vi "Teleop.vi"(10 "Match Info":T1={"Autonomous Elapsed Seconds"=0.0, "TeleOp Elapsed Seconds"=0.0, "Disabled Elapsed Seconds"=0.0, "Visited Autonomous"=FALSE, "Visited TeleOp"=FALSE, "Visited Disabled"=FALSE, "Autonomous Settings"={"Autonomous Style"=enum."Independent", "VI Refnum"=refnum}}, 11 "Call Context":T2) -> ()   [LabVIEW 2011]
doc: "This VI is called for each TeleOp packet received from the DS where the robot is not disabled. It is often used to read from the joysticks and update I/O or to update setpoints for timed control loops. It should complete and return within 20 milliseconds or it may miss DS packets."
uses:
  <vilib>/Rock Robotics/WPI/DriverStation/WPI_DriverStationDerivedRobotMode.ctl
  <vilib>/Rock Robotics/WPI/DriverStation/WPI_DriverStationMatch Info.ctl
  <vilib>/Rock Robotics/WPI/Relay/WPI_RelayValue.ctl
  <vilib>/Rock Robotics/WPI/DriverStation/DriverStationLCD/WPI_DriverStationLCDLCDLine.ctl
  Robot Global Data.vi
panel:
  in  "LDrive0":dbl
  in  "Rdrive0":dbl=0.9
  in  "Rdrive2":dbl=0.6
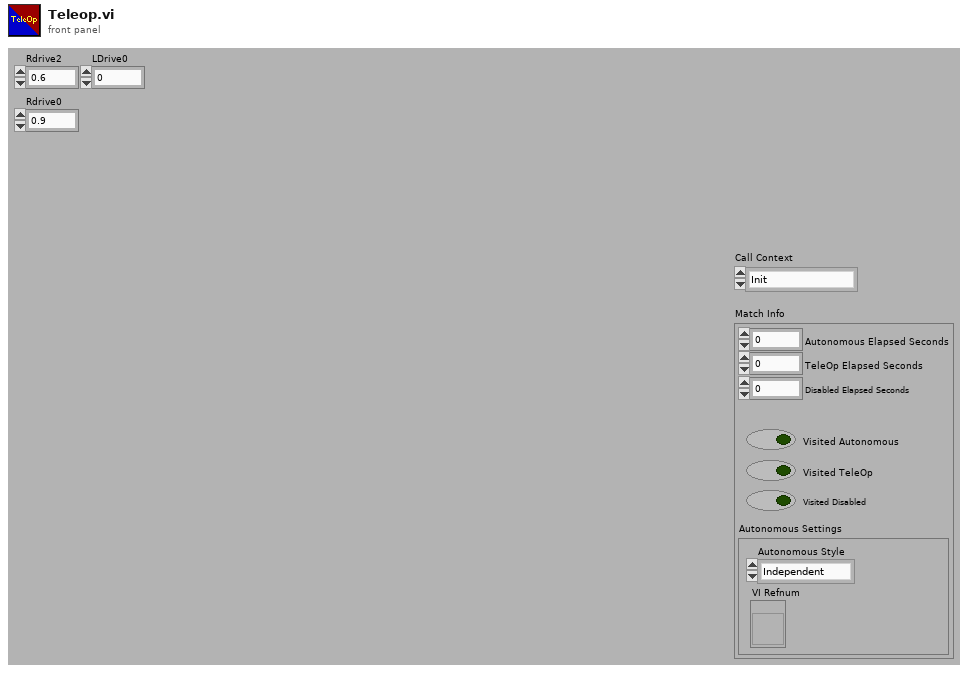
[diagram p1: front panel]
types:
  T1 = typedef "WPI_DriverStationMatch Info.ctl" = cluster{"Autonomous Elapsed Seconds":dbl, "TeleOp Elapsed Seconds":dbl, "Disabled Elapsed Seconds":dbl, "Visited Autonomous":bool, "Visited TeleOp":bool, "Visited Disabled":bool, "Autonomous Settings":cluster{"Autonomous Style":enum16{"Iterative", "Independent"}, "VI Refnum":refnum<vi>}}
  T2 = typedef "WPI_DriverStationDerivedRobotMode.ctl" = enum16{"Init", "Execute", "Stop"}
  T3 = typedef "WPI_RelayValue.ctl" = enum16{"Off", "On", "Forward", "Reverse"}
  T4 = typedef "WPI_JoystickDevRef.ctl" = cluster{"Device":T5}
  T5 = typedef "WPI_JoystickDeviceEnum.ctl" = enum16{"USB 1", "USB 2", "USB 3", "USB 4", "Kinect 1", "Kinect 2"}
  T6 = typedef "WPI_JoystickButtonState.ctl" = cluster{"Button 1":bool, "Button 2":bool, "Button 3":bool, "Button 4":bool, "Button 5":bool, "Button 6":bool, "Button 7":bool, "Button 8":bool, "Button 9":bool, "Button 10":bool, "Button 11":bool, "Button 12":bool}
  T7 = cluster{"axis 1 (x)":dbl, "axis 2 (y)":dbl, "axis 3 (throttle)":dbl, "axis 4":dbl, "axis 5":dbl, "axis 6":dbl}
  T8 = typedef "WPI_MotorControlDeviceRef.ctl" = cluster{"DeviceStatus":errorcluster, "Type":enum16{"PWM", "CAN"}, "PWM":cluster{"Digital Module":T9, "PWM Channel":T10, "DeadBand":T11}, "CAN":cluster{"Device Number":u8, "Control Mode":T12, "Semaphore":T13, "Max Vout":dbl}, "Invert":bool, "TransformRef":T14, "InvTransformRef":T14}
  T9 = typedef "FPGA_TypedefDigitalModule.ctl" = enum16{"Digital Module 1", "Digital Module 2"}
  T10 = typedef "FPGA_DIOPWMChannel.ctl" = enum8{"PWM 1", "PWM 2", "PWM 3", "PWM 4", "PWM 5", "PWM 6", "PWM 7", "PWM 8", "PWM 9", "PWM 10", "Invalid"}
  T11 = typedef "WPI_PWMDeadband.ctl" = cluster{"Name":string, "maxPositivePwm":i32, "minPositivePwm":i32, "centerPwm":i32, "maxNegativePwm":i32, "minNegativePwm":i32, "angularRange":u16}
  T12 = typedef "WPI_CANJaguar_ControlMode.ctl" = enum8{"Percent VBus", "Current", "Speed", "Position", "Voltage"}
  T13 = typedef "Semaphore RefNum" = refnum<k1>
  T14 = typedef "WPI_PWMTransform_ConPane.ctl" = refnum<vi>
  T15 = cluster{"Driver Station Digital Input (1-8)[0]":bool, "Driver Station Digital Input (1-8)[1]":bool, "Driver Station Digital Input (1-8)[2]":bool, "Driver Station Digital Input (1-8)[3]":bool, "Driver Station Digital Input (1-8)[4]":bool, "Driver Station Digital Input (1-8)[5]":bool, "Driver Station Digital Input (1-8)[6]":bool, "Driver Station Digital Input (1-8)[7]":bool, "Driver Station Digital Input (1-8)[8]":bool}
  T16 = typedef "WPI_RelayDevRef.ctl" = cluster{"DevStatus":errorcluster, "Relay Channel":T17, "Digital Module":T9, "Relay Direction":T18}
  T17 = typedef "FPGA_DIORelayChannel.ctl" = enum8{"Relay 1", "Relay 2", "Relay 3", "Relay 4", "Relay 5", "Relay 6", "Relay 7", "Relay 8", "Invalid"}
  T18 = typedef "WPI_RelayDirection.ctl" = enum16{"Both directions", "Forward only", "Reverse only"}
  T19 = typedef "WPI_DigitalInputDevRef.ctl" = cluster{"DevStatus":errorcluster, "DIO Channel":T20, "Digital Module":T9}
  T20 = typedef "FPGA_DIOChannel.ctl" = enum8{"DIO 1", "DIO 2", "DIO 3", "DIO 4", "DIO 5", "DIO 6", "DIO 7", "DIO 8", "DIO 9", "DIO 10", "DIO 11", "DIO 12", "DIO 13", "DIO 14", "Invalid"}
  T21 = typedef "WPI_EncoderDevRef.ctl" = cluster{"DevStatus":errorcluster, "EncoderIndex":T22, "CounterIndex":T23, "DistancePerCount":dbl, "Decoding Type":T24}
  T22 = typedef "FPGA_EncoderIdx.ctl" = enum8{"Enc 0", "Enc 1", "Enc 2", "Enc 3", "Invalid"}
  T23 = typedef "FPGA_CounterCtrSystemIndex.ctl" = enum8{"Ctr 0", "Ctr 1", "Ctr 2", "Ctr 3", "Ctr 4", "Ctr 5", "Ctr 6", "Ctr 7", "Invalid"}
  T24 = typedef "WPI_EncoderType.ctl" = enum16{"1x", "2x", "4x"}
  T25 = typedef "WPI_DriverStationLCDLCDLine.ctl" = enum16{"Main - Line 1", "User - Line 2", "User - Line 3", "User - Line 4", "User - Line 5", "User - Line 6"}
  T26 = typedef "WPI_ServoDeviceRef.ctl" = cluster{"DeviceStatus":errorcluster, "Digital Module":T9, "PWM Channel":T10, "DeadBand":T11}
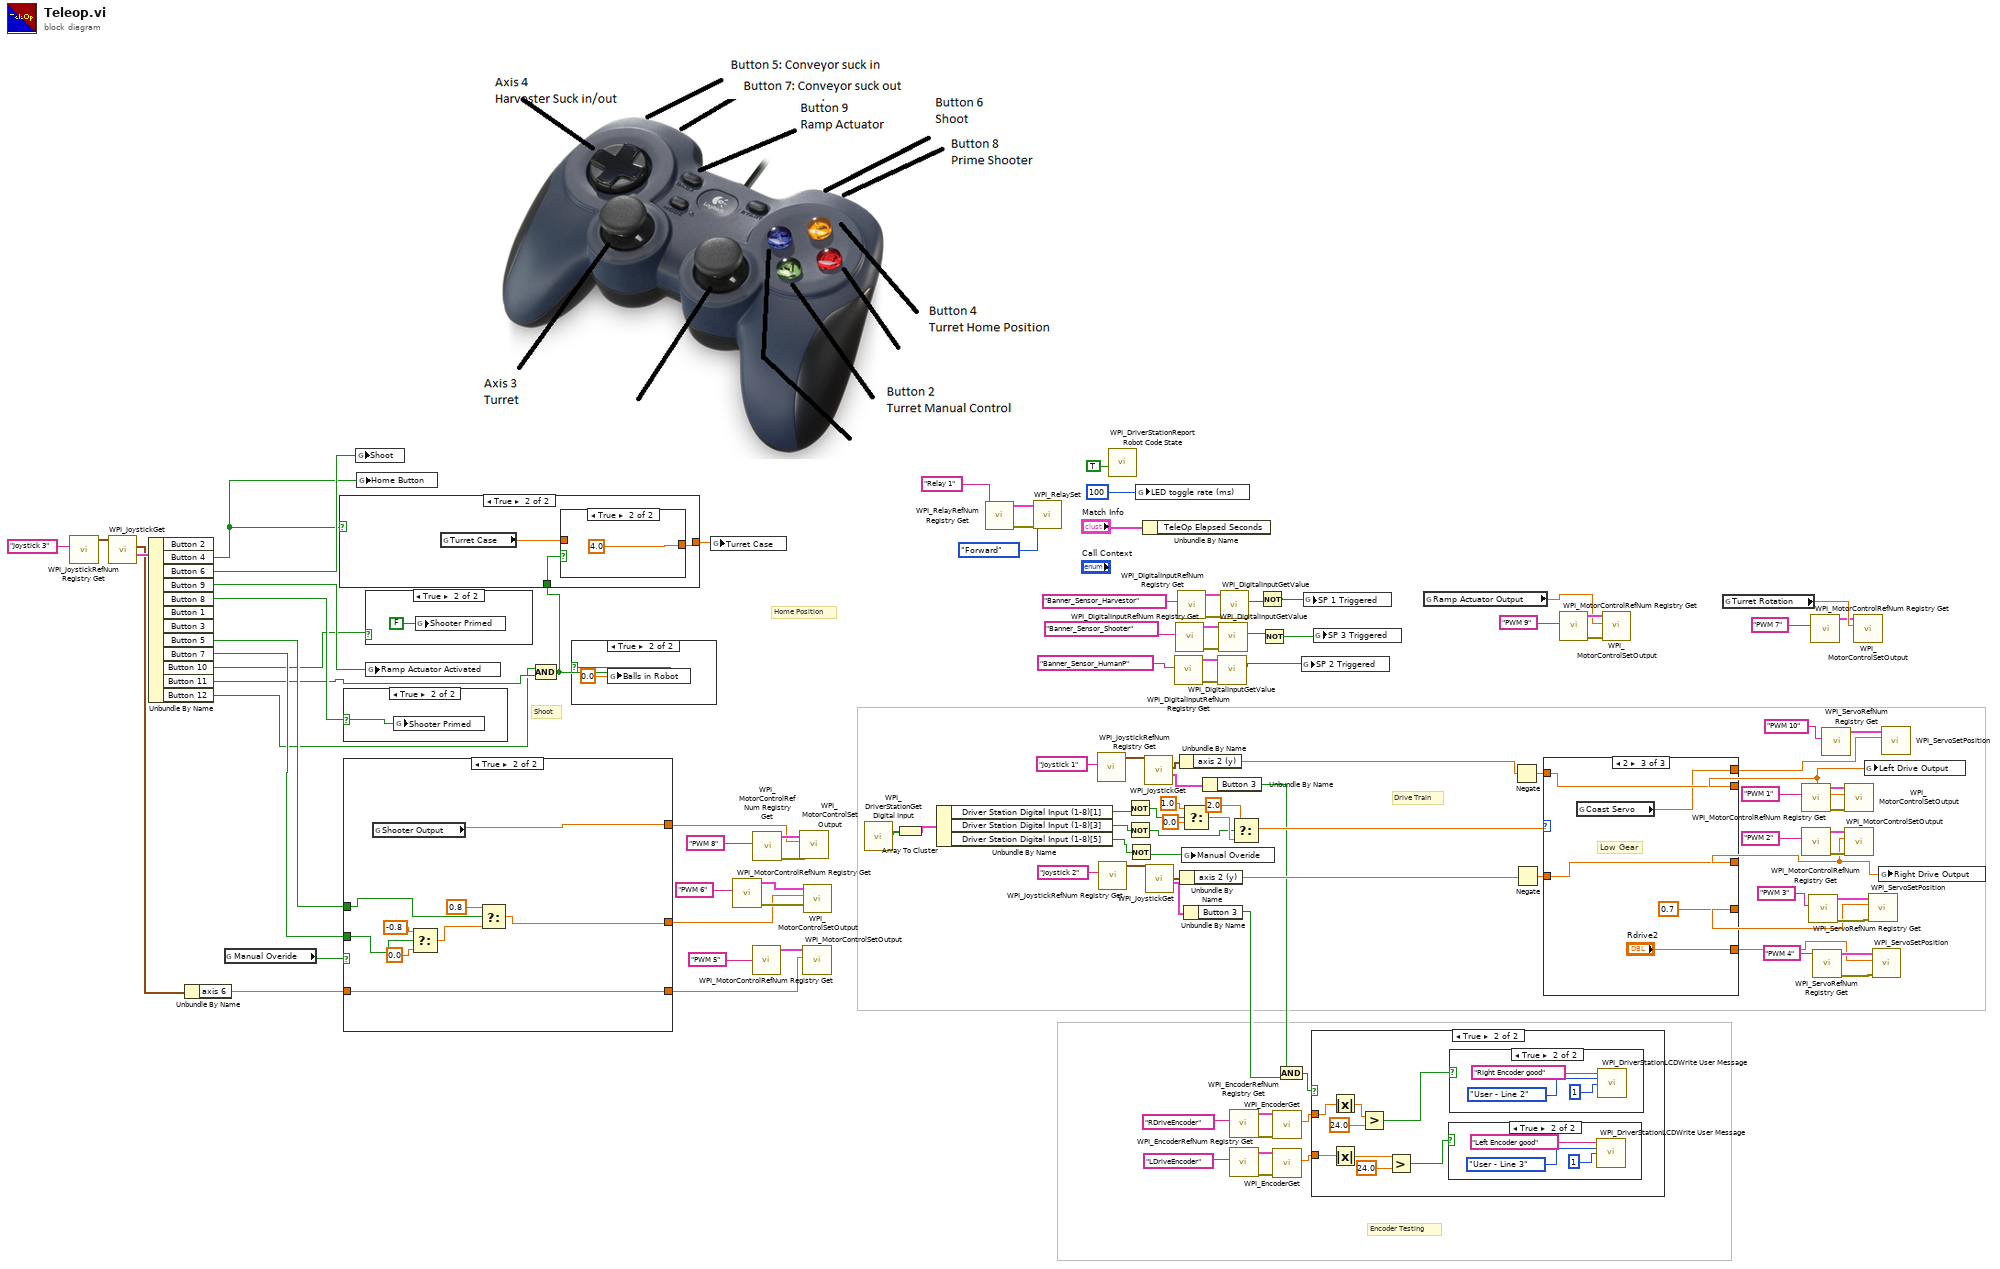
[diagram p0: block diagram]
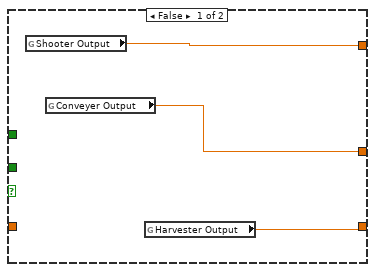
[diagram p7: hidden frame]
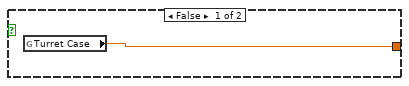
[diagram p9: hidden frame]
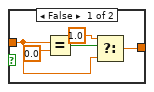
[diagram p10: hidden frame]
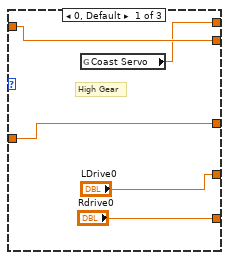
[diagram p11: hidden frame]
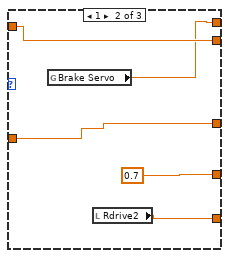
[diagram p12: hidden frame]
diagram:
  # "Encoder Testing"
  # "Shoot"
  # "Home Position"
  # "Drive Train"
  n1 = call <vilib>:"WPI_JoystickRefNum Registry Get.vi"("refnum name"="Joystick 3") -> ("JoystickDevRef"=w64:T4)  [unwired: 9 in, 1 out]
  n2 = call <vilib>:"WPI_JoystickGet.vi"("JoystickDevRef"=w64) -> ("Buttons"=w65:T6, "Axes"=w38:T7)  [unwired: 4 in, 1 out]
  n3 = Unbundle By Name(w65) -> ("Button 4"=w25:bool, "Button 6"=w63:bool, "Button 9"=w67:bool, "Button 8"=w39:bool, "Button 5"=w33:bool, "Button 7"=w32:bool, "Button 10"=w24:bool, "Button 11"=w23:bool, "Button 12"=w22:bool)  [unwired: 3 out]
  n4 = Unbundle By Name(w38) -> ("axis 6"=w20:dbl)
  n5 = global read "Robot Global Data.vi" "Manual Overide"() -> (w27:bool)
  n6 = case shown="True" w39 {
    selector: w39 -> [_ w112]
    frame False {
    }
    frame True {
      n7 = global write "Robot Global Data.vi" "Shooter Primed"(w112) -> ()
    }
  }
  n8 = case shown="True" w27 {
    tunnel: [w115 w116] -> w34
    tunnel: w33 -> [_ w119]
    tunnel: w32 -> [_ w120]
    tunnel: [w114 w118] -> w28
    tunnel: [w113 w117] -> w21
    tunnel: w20 -> [_ w117]
    frame False {
      n9 = global read "Robot Global Data.vi" "Shooter Output"() -> (w115:dbl)
      n10 = global read "Robot Global Data.vi" "Conveyer Output"() -> (w114:dbl)
      n11 = global read "Robot Global Data.vi" "Harvester Output"() -> (w113:dbl)
    }
    frame True {
      n12 = global read "Robot Global Data.vi" "Shooter Output"() -> (w116:dbl)
      n13 = Select(t=-0.8, s=w120, f=0.0) -> (s? t:f=w124:dbl)
      n14 = Select(t=0.8, s=w119, f=w124) -> (s? t:f=w118:dbl)
    }
  }
  n15 = global write "Robot Global Data.vi" "Shoot"(w63) -> ()
  n16 = global write "Robot Global Data.vi" "Home Button"(w25) -> ()
  n17 = case shown="True" w24 {
    frame False {
    }
    frame True {
      n18 = global write "Robot Global Data.vi" "Shooter Primed"(FALSE ("Shooter Primed")) -> ()
    }
  }
  n19 = global write "Robot Global Data.vi" "Ramp Actuator Activated"(w67) -> ()
  n20 = Compound Arithmetic op=AND(w22, w23) -> (w19:bool)
  n21 = case shown="True" w25 {
    tunnel: [w126 w127] -> w18
    tunnel: w19 -> [_ w129]
    frame False {
      n22 = global read "Robot Global Data.vi" "Turret Case"() -> (w126:dbl)
    }
    frame True {
      n23 = global read "Robot Global Data.vi" "Turret Case"() -> (w128:dbl)
      n24 = case shown="True" w129 {
        tunnel: w128 -> [w131 _]
        tunnel: [w130 4.0 ("Turret Case")] -> w127
        frame False {
          n25 = Equal?(x=w131, y=0.0) -> (x = y?=w133:bool)
          n26 = Select(t=1.0, s=w133, f=w131) -> (s? t:f=w130:dbl)
        }
        frame True {
        }
      }
    }
  }
  n27 = case shown="True" w19 {
    frame False {
    }
    frame True {
      n28 = global write "Robot Global Data.vi" "Balls in Robot"(0.0 ("Balls in Robot")) -> ()
    }
  }
  n29 = global write "Robot Global Data.vi" "Turret Case"(w18) -> ()
  n30 = call <vilib>:"WPI_MotorControlRefNum Registry Get.vi"("refnum name"="PWM 6") -> ("error out"=w29:errorcluster, "MotorControlDevRef"=w30:T8)  [unwired: 9 in]
  n31 = call <vilib>:"WPI_MotorControlRefNum Registry Get.vi"("refnum name"="PWM 5") -> ("MotorControlDevRef"=w57:T8)  [unwired: 9 in, 1 out]
  n32 = call <vilib>:"WPI_MotorControlRefNum Registry Get.vi"("refnum name"="PWM 8") -> ("error out"=w41:errorcluster, "MotorControlDevRef"=w42:T8)  [unwired: 9 in]
  n33 = call <vilib>:"WPI_MotorControlSetOutput.vi"("error in (no error)"=w41, "Output"=w34, "MotorControlDevRef"=w42) -> ()  [unwired: 7 in, 2 out]
  n34 = call <vilib>:"WPI_MotorControlSetOutput.vi"("Output"=w21, "MotorControlDevRef"=w57) -> ()  [unwired: 8 in, 2 out]
  n35 = call <vilib>:"WPI_MotorControlSetOutput.vi"("error in (no error)"=w29, "Output"=w28, "MotorControlDevRef"=w30) -> ()  [unwired: 7 in, 2 out]
  n36 = call <vilib>:"WPI_DriverStationGet Digital Input.vi"() -> ("Driver Station Digital Input (1-8)"=w86:bool[])  [unwired: 11 in]
  n37 = Array To Cluster(array=w86) -> (cluster=w108:T15)
  n38 = Unbundle By Name(w108) -> ("Driver Station Digital Input (1-8)[1]"=w89:bool, "Driver Station Digital Input (1-8)[3]"=w88:bool, "Driver Station Digital Input (1-8)[5]"=w35:bool)
  n39 = call <vilib>:"WPI_RelayRefNum Registry Get.vi"("refnum name"="Relay 1") -> ("error out"=w61:errorcluster, "RelayDevRef"=w62:T16)  [unwired: 9 in]
  n40 = call <vilib>:"WPI_RelaySet.vi"("error in (no error)"=w61, "RelayValue"=WPI_RelayValue."Forward", "RelayDevRef"=w62) -> ()  [unwired: 7 in, 2 out]
  n41 = call <vilib>:"WPI_JoystickRefNum Registry Get.vi"("refnum name"="Joystick 1") -> ("JoystickDevRef"=w101:T4)  [unwired: 9 in, 1 out]
  n42 = call <vilib>:"WPI_JoystickRefNum Registry Get.vi"("refnum name"="Joystick 2") -> ("JoystickDevRef"=w99:T4)  [unwired: 9 in, 1 out]
  n43 = call <vilib>:"WPI_DriverStationReport Robot Code State.vi"("TeleOp"=TRUE ("Autonomous")) -> ()  [unwired: 10 in, 1 out]
  n44 = Not(x=w89) -> (.not. x?=w87:bool)
  n45 = Not(x=w88) -> (.not. x?=w37:bool)
  n46 = Not(x=w35) -> (.not. x?=w36:bool)
  n47 = global write "Robot Global Data.vi" "LED toggle rate (ms)"(u32 100 ("LED ms toggle rate")) -> ()
  n48 = Unbundle By Name("Match Info") -> ()  [unwired: 1 out]
  n49 = call <vilib>:"WPI_JoystickGet.vi"("JoystickDevRef"=w101) -> ("Buttons"=w15:T6, "Axes"=w16:T7)  [unwired: 4 in, 1 out]
  n50 = call <vilib>:"WPI_JoystickGet.vi"("JoystickDevRef"=w99) -> ("Buttons"=w17:T6, "Axes"=w100:T7)  [unwired: 4 in, 1 out]
  n51 = call <vilib>:"WPI_DigitalInputRefNum Registry Get.vi"("refnum name"="Banner_Sensor_HumanP") -> ("error out"=w52:errorcluster, "DigitalInputDevRef"=w51:T19)  [unwired: 9 in]
  n52 = call <vilib>:"WPI_DigitalInputRefNum Registry Get.vi"("refnum name"="Banner_Sensor_Shooter") -> ("error out"=w53:errorcluster, "DigitalInputDevRef"=w54:T19)  [unwired: 9 in]
  n53 = call <vilib>:"WPI_DigitalInputRefNum Registry Get.vi"("refnum name"="Banner_Sensor_Harvestor") -> ("error out"=w56:errorcluster, "DigitalInputDevRef"=w55:T19)  [unwired: 9 in]
  n54 = Unbundle By Name(w16) -> ("axis 2 (y)"=w85:dbl)
  n55 = Unbundle By Name(w100) -> ("axis 2 (y)"=w83:dbl)
  n56 = Select(t=1.0, s=w87, f=0.0 ("t")) -> (s? t:f=w105:dbl)
  n57 = global write "Robot Global Data.vi" "Manual Overide"(w36) -> ()
  n58 = Unbundle By Name(w17) -> ("Button 3"=w13:bool)
  n59 = Unbundle By Name(w15) -> ("Button 3"=w14:bool)
  n60 = call <vilib>:"WPI_DigitalInputGetValue.vi"("error in (no error)"=w52, "DigitalInputDevRef"=w51) -> ("Value"=w47:bool)  [unwired: 7 in, 2 out]
  n61 = call <vilib>:"WPI_DigitalInputGetValue.vi"("error in (no error)"=w53, "DigitalInputDevRef"=w54) -> ("Value"=w46:bool)  [unwired: 7 in, 2 out]
  n62 = call <vilib>:"WPI_DigitalInputGetValue.vi"("error in (no error)"=w56, "DigitalInputDevRef"=w55) -> ("Value"=w44:bool)  [unwired: 7 in, 2 out]
  n63 = call <vilib>:"WPI_EncoderRefNum Registry Get.vi"("refnum name"="RDriveEncoder") -> ("error out"=w9:errorcluster, "EncoderDevRef"=w10:T21)  [unwired: 9 in]
  n64 = call <vilib>:"WPI_EncoderRefNum Registry Get.vi"("refnum name"="LDriveEncoder") -> ("error out"=w8:errorcluster, "EncoderDevRef"=w7:T21)  [unwired: 9 in]
  n65 = Select(t=2.0, s=w37, f=w105) -> (s? t:f=w103:dbl)
  n66 = Not(x=w44) -> (.not. x?=w43:bool)
  n67 = Not(x=w46) -> (.not. x?=w45:bool)
  n68 = call <vilib>:"WPI_EncoderGet.vi"("error in (no error)"=w9, "EncoderDevRef"=w10) -> ("Distance"=w5:dbl)  [unwired: 4 in, 5 out]
  n69 = call <vilib>:"WPI_EncoderGet.vi"("error in (no error)"=w8, "EncoderDevRef"=w7) -> ("Distance"=w4:dbl)  [unwired: 4 in, 5 out]
  n70 = And(x=w14, y=w13) -> (x .and. y?=w12:bool)
  n71 = global write "Robot Global Data.vi" "SP 2 Triggered"(w47) -> ()
  n72 = global write "Robot Global Data.vi" "SP 1 Triggered"(w43) -> ()
  n73 = case shown="True" w12 {
    tunnel: w5 -> [_ w139]
    tunnel: w4 -> [_ w138]
    frame False {
    }
    frame True {
      n74 = Absolute Value(x=w139) -> (abs(x)=w140:dbl)
      n75 = Absolute Value(x=w138) -> (abs(x)=w137:dbl)
      n76 = Greater?(x=w140, y=24.0) -> (0:w143:bool)
      n77 = Greater?(x=w137, y=24.0) -> (0:w141:bool)
      n78 = case shown="True" w141 {
        frame False {
        }
        frame True {
          n79 = call <vilib>:"WPI_DriverStationLCDWrite User Message.vi"("line text"="Left Encoder good", "line"=WPI_DriverStationLCDLCDLine."User - Line 3", "starting column"=i8 1) -> ()  [unwired: 2 in, 11 out]
        }
      }
      n80 = case shown="True" w143 {
        frame False {
        }
        frame True {
          n81 = call <vilib>:"WPI_DriverStationLCDWrite User Message.vi"("line text"="Right Encoder good", "line"=WPI_DriverStationLCDLCDLine."User - Line 2", "starting column"=i8 1) -> ()  [unwired: 2 in, 11 out]
        }
      }
    }
  }
  n82 = global write "Robot Global Data.vi" "SP 3 Triggered"(w45) -> ()
  n83 = global read "Robot Global Data.vi" "Ramp Actuator Output"() -> (w26:dbl)
  n84 = Negate(x=w85) -> (-x=w84:dbl)
  n85 = Negate(x=w83) -> (-x=w82:dbl)
  n86 = case shown="2" w103 {
    tunnel: w82 -> [w155 w158 w165]
    tunnel: [w155 w158 w165] -> w74
    tunnel: [w154 w157 w164] -> w75
    tunnel: ["LDrive0" 0.7 0.7] -> w91
    tunnel: ["Rdrive0" w159 "Rdrive2"] -> w90
    tunnel: w84 -> [w154 w157 w164]
    tunnel: [w151 w156 w161] -> w1
    frame 0, Default {
      # "High Gear"
      n87 = global read "Robot Global Data.vi" "Coast Servo"() -> (w151:dbl)
    }
    frame 1 {
      n88 = global read "Robot Global Data.vi" "Brake Servo"() -> (w156:dbl)
      n89 = local read "Rdrive2"() -> (w159:dbl)
    }
    frame 2 {
      # "Low Gear"
      n90 = global read "Robot Global Data.vi" "Coast Servo"() -> (w161:dbl)
    }
  }
  n91 = call <vilib>:"WPI_MotorControlRefNum Registry Get.vi"("refnum name"="PWM 9") -> ("error out"=w72:errorcluster, "MotorControlDevRef"=w71:T8)  [unwired: 9 in]
  n92 = call <vilib>:"WPI_MotorControlSetOutput.vi"("error in (no error)"=w72, "Output"=w26, "MotorControlDevRef"=w71) -> ()  [unwired: 7 in, 2 out]
  n93 = global read "Robot Global Data.vi" "Turret Rotation"() -> (w70:dbl)
  n94 = call <vilib>:"WPI_MotorControlRefNum Registry Get.vi"("refnum name"="PWM 1") -> ("error out"=w79:errorcluster, "MotorControlDevRef"=w81:T8)  [unwired: 9 in]
  n95 = call <vilib>:"WPI_MotorControlRefNum Registry Get.vi"("refnum name"="PWM 2") -> ("error out"=w78:errorcluster, "MotorControlDevRef"=w77:T8)  [unwired: 9 in]
  n96 = call <vilib>:"WPI_ServoRefNum Registry Get.vi"("refnum name"="PWM 3") -> ("error out"=w95:errorcluster, "ServoDeviceRef"=w96:T26)  [unwired: 9 in]
  n97 = call <vilib>:"WPI_MotorControlRefNum Registry Get.vi"("refnum name"="PWM 7") -> ("MotorControlDevRef"=w68:T8)  [unwired: 9 in, 1 out]
  n98 = call <vilib>:"WPI_ServoRefNum Registry Get.vi"("refnum name"="PWM 4") -> ("error out"=w94:errorcluster, "ServoDeviceRef"=w93:T26)  [unwired: 9 in]
  n99 = call <vilib>:"WPI_ServoRefNum Registry Get.vi"("refnum name"="PWM 10") -> ("ServoDeviceRef"=w3:T26)  [unwired: 9 in, 1 out]
  n100 = call <vilib>:"WPI_MotorControlSetOutput.vi"("error in (no error)"=w79, "Output"=w75, "MotorControlDevRef"=w81) -> ()  [unwired: 7 in, 2 out]
  n101 = call <vilib>:"WPI_MotorControlSetOutput.vi"("error in (no error)"=w78, "Output"=w74, "MotorControlDevRef"=w77) -> ()  [unwired: 7 in, 2 out]
  n102 = call <vilib>:"WPI_MotorControlSetOutput.vi"("Output"=w70, "MotorControlDevRef"=w68) -> ()  [unwired: 8 in, 2 out]
  n103 = global write "Robot Global Data.vi" "Left Drive Output"(w75) -> ()
  n104 = call <vilib>:"WPI_ServoSetPosition.vi"("error in (no error)"=w95, "Position"=w91, "ServoDeviceRef"=w96) -> ()  [unwired: 7 in, 2 out]
  n105 = call <vilib>:"WPI_ServoSetPosition.vi"("error in (no error)"=w94, "Position"=w90, "ServoDeviceRef"=w93) -> ()  [unwired: 7 in, 2 out]
  n106 = global write "Robot Global Data.vi" "Right Drive Output"(w74) -> ()
  n107 = call <vilib>:"WPI_ServoSetPosition.vi"("Position"=w1, "ServoDeviceRef"=w3) -> ()  [unwired: 8 in, 2 out]
